vi "Verify File or Folder Exist.vi"(0 "path":path) -> (14 "dup path":path, 17 "file or folder exists?":bool, 19 "Path Type":enum16{"unknown", "File", "Folder"}(ring))   [LabVIEW 2020, in "Generic Utilities.lvclass"]
uses:
  Generic Utilities.lvclass
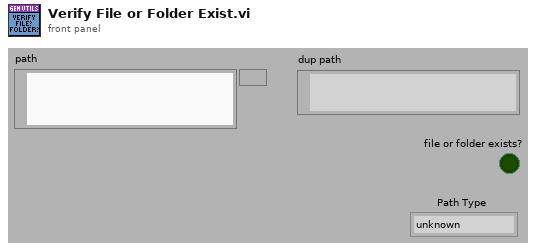
[diagram p1: front panel]
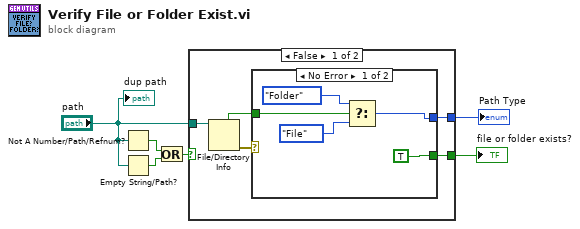
[diagram p0: block diagram]
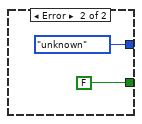
[diagram p2: hidden frame]
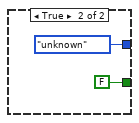
[diagram p3: hidden frame]
diagram:
  n1 = Not A Number/Path/Refnum?(number/path/refnum="path") -> (NaN/Path/Refnum?=w1:bool)
  n2 = Empty String/Path?(string/path="path") -> (empty?=w2:bool)
  n3 = Or(x=w1, y=w2) -> (x .or. y?=w3:bool)
  n4 = case shown="False" w3 {
    tunnel: [w9 FALSE] -> w5
    tunnel: "path" -> [w11 _]
    tunnel: [w8 enum16{"unknown", "File", "Folder"}."unknown" ("Path Type")] -> w6
    frame False {
      n5 = File/Directory Info(path=w11) -> (directory=w7:bool, error out=w10:errorcluster)  [unwired: 1 in, 5 out]
      n6 = case shown="No Error" w10 {
        tunnel: [TRUE FALSE] -> w9
        tunnel: [w12 enum16{"unknown", "File", "Folder"}."unknown" ("Path Type")] -> w8
        tunnel: w7 -> [w15 _]
        frame No Error {
          n7 = Select(t=enum16{"unknown", "File", "Folder"}."Folder" ("Path Type"), s=w15, f=enum16{"unknown", "File", "Folder"}."File" ("Path Type")) -> (s? t:f=w12:enum16{"unknown", "File", "Folder"})
        }
        frame Error {
        }
      }
    }
    frame True {
    }
  }
  "file or folder exists?" <- w5
  "Path Type" <- w6
  "dup path" <- "path"
